vi "Sort_Array_Indicies.vi"(0 "unsorted array":dbl[](array[numeric]) format="%.2f") -> (1 "sorted array":dbl[](array[numeric]) format="%.2f", 2 "Sort Index":i32[](array[numeric]))   [LabVIEW 2020]
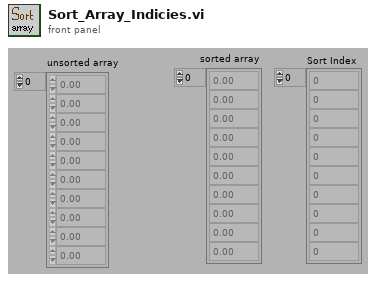
[diagram p1: front panel]
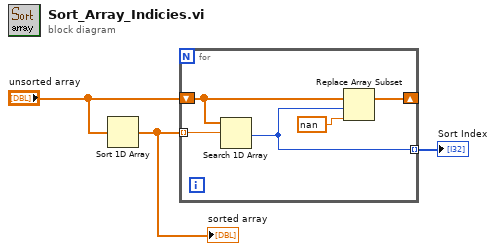
[diagram p0: block diagram]
diagram:
  n1 = Sort 1D Array(array="unsorted array") -> (sorted array=w2:dbl[])
  "sorted array" <- w2
  n2 = for {
    tunnel: w2 -> [w8] mode=indexing
    shift-right: [w6] -> _
    shift-left: "unsorted array" -> [w7]
    tunnel: [w4] -> w1 mode=indexing
    n3 = Search 1D Array(1D array=w7, element=w8) -> (index of element=w4:i32)  [unwired: 1 out]
    n4 = Replace Array Subset(array=w7, new element=nan ("new element/subarray"), index=w4) -> (w6:dbl[])
  }
  "Sort Index" <- w1
